vi "init.vi"(0 "DynamicFrameBuilder in":refnum<class "DynamicFrameBuilder.lvclass">, 5 "Address":u8, 7 "Function":u8, 9 "DataSize":i32, 11 "error in (no error)":errorcluster) -> (4 "DynamicFrameBuilder out":refnum<class "DynamicFrameBuilder.lvclass">, 15 "error out":errorcluster)   [LabVIEW 2015, in "RTModbus.lvlib" / "DynamicFrameBuilder.lvclass"]
uses:
  DynamicFrameBuilder.lvclass
  DynamicFrameBuilder.lvclass/DynamicFrameBuilder.ctl
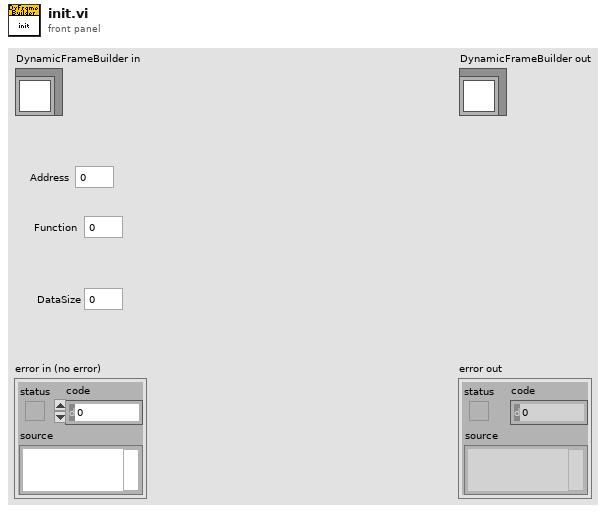
[diagram p1: front panel]
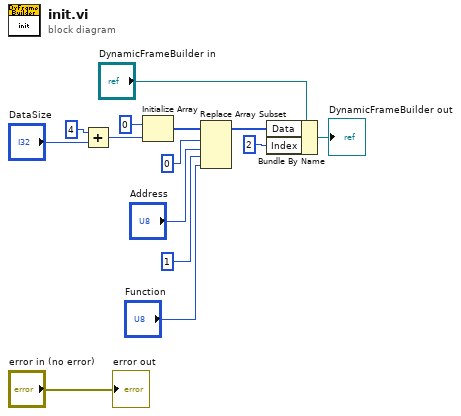
[diagram p0: block diagram]
diagram:
  n1 = Add(x=4, y="DataSize") -> (x+y=w12:i32)
  n2 = Initialize Array(u8 0 ("element"), w12) -> (w14:u8[])
  n3 = Replace Array Subset(array=w14, new element #1="Address", index #1=0 ("index"), new element #2="Function", index #2=1 ("index")) -> (w3:u8[])
  n4 = Bundle By Name(cluster="DynamicFrameBuilder in", "Data"=w3, "Index"=2) -> (→"DynamicFrameBuilder out":refnum<class "DynamicFrameBuilder.lvclass">)
  "error out" <- "error in (no error)"
